vi "display_subVI.vi"(11 "input cluster":T2={"path to binary file"=path "C:/Users/Lenovo/Desktop/szakdoga/data", "Start Cursor"=timestamp(0 s since 1904-01-01), "Sec"=60.0, "crossing level"=0.0, "threshold"=0.35, "avg window size"=5, "peak detect width"=30, "invert"=FALSE, "SNR window width [Hz]"=0.5, "felharmonikus N"=2, "End cursor"=timestamp(0 s since 1904-01-01)} {"peak detect width" min=3; "threshold" format="%0.2f"}) -> (3 "data cluster":T1)   [LabVIEW 2019]
uses:
  <vilib>/Waveform/WDTOps.llb/WDT Get Waveform Subset DBL.vi
  <vilib>/Analysis/NI_AALBase.lvlib
  <vilib>/Analysis/1siggen.llb/Ramp Pattern by Samples.vi
  <vilib>/Analysis/1siggen.llb/Ramp Pattern by Delta.vi
panel:
  out "Z axis SNR":cluster{"Ramp Pattern":dbl[], dbl[]}[](graph)
  out "Y axis SNR":cluster{"Ramp Pattern":dbl[], dbl[]}[](graph)
  out "X axis SNR":cluster{"Ramp Pattern":dbl[], dbl[]}[](graph)
  out "resultant SNR":cluster{"Ramp Pattern":dbl[], dbl[]}[](graph)
  out "SNR":dbl
  out "csapás impulzus":cluster{"Ramp Pattern":dbl[], dbl[]}(graph)
  out "csapásszám":cluster{"Ramp Pattern":dbl[], dbl[]}[](graph)
  in  "felbontás [s]":dbl=20.0
  out "freq [Hz]":dbl
  out "PSD":cluster{"f0":dbl, "df":dbl, "magnitude":dbl[]}[](graph)
  out "inspection":cluster{"Y":dbl[], "Y":dbl[]}[](graph)
  out "inspected section":waveform(dbl)[](graph)
  out "read in data":waveform(dbl)[](graph)
  # "30mp-es ablakokkal számított SNR meta adatok"
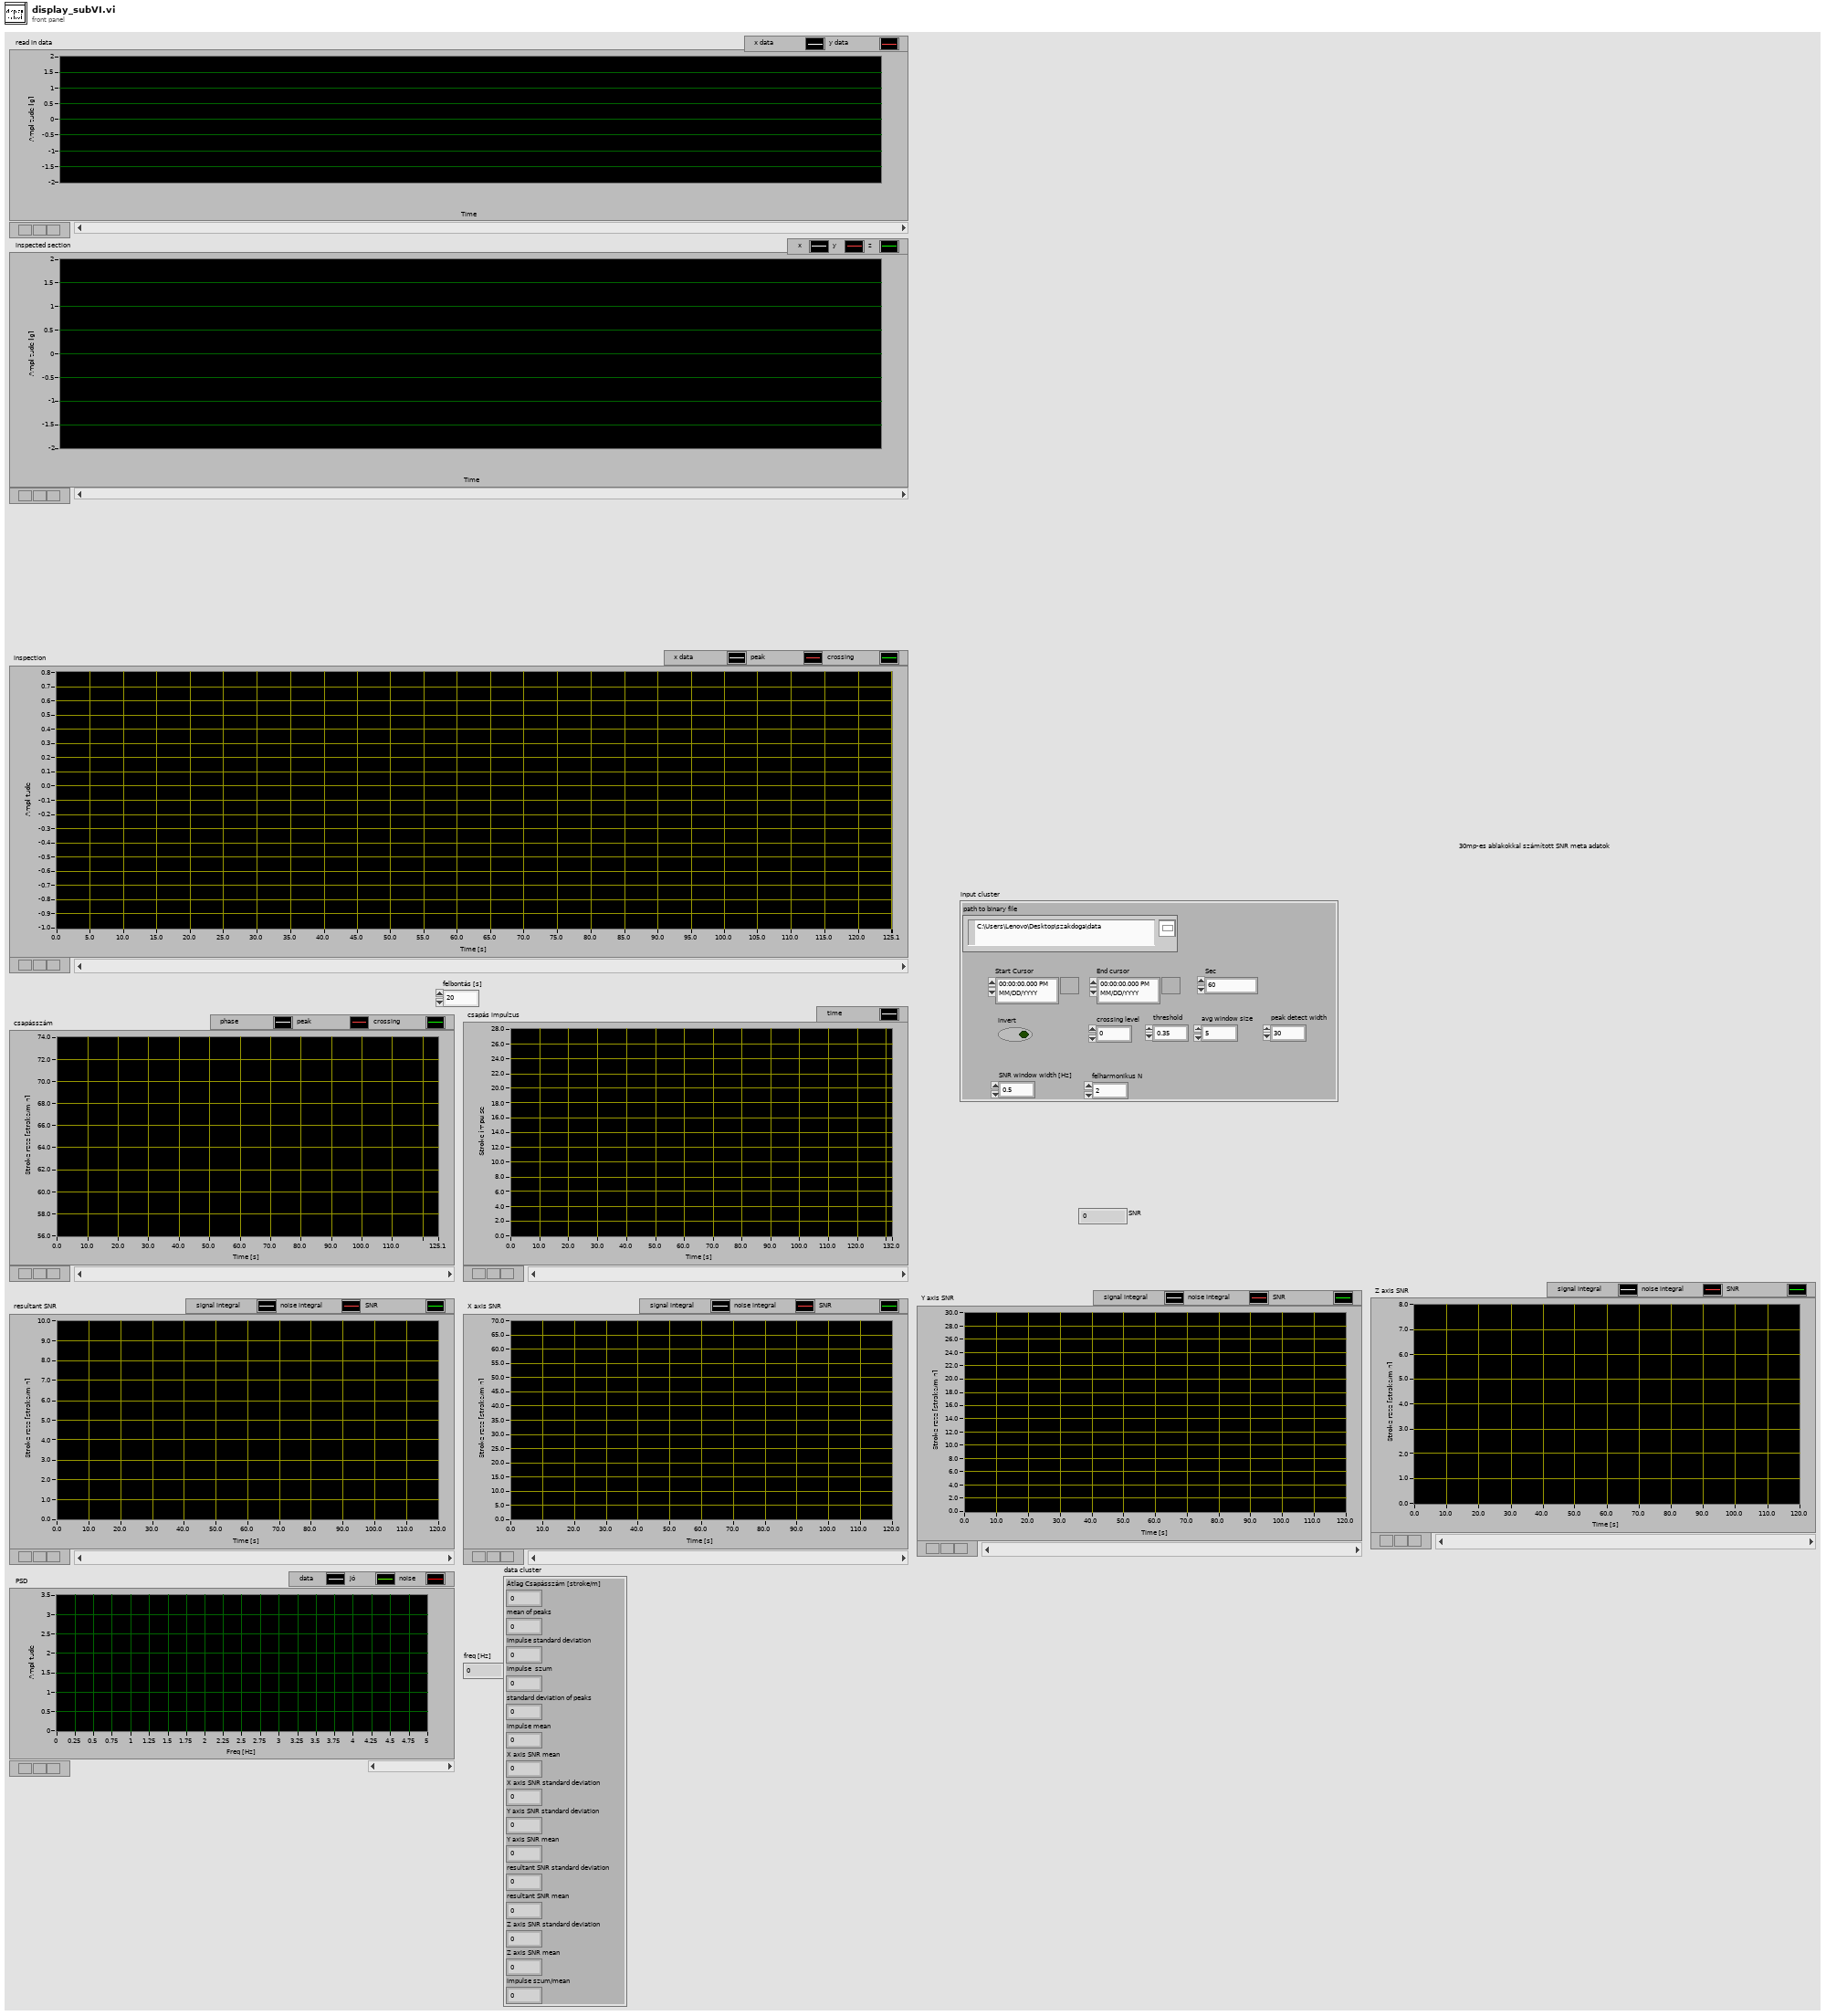
[diagram p1: front panel]
types:
  T1 = cluster{"Átlag Csapásszám [stroke/m]":dbl, "mean of peaks":dbl, "impulse standard deviation":dbl, "impulse  szum":dbl, "standard deviation of peaks":dbl, "impulse mean":dbl, "X axis SNR mean":dbl, "X axis SNR standard deviation":dbl, "Y axis SNR standard deviation":dbl, "Y axis SNR mean":dbl, "resultant SNR standard deviation":dbl, "resultant SNR mean":dbl, "Z axis SNR standard deviation":dbl, "Z axis SNR mean":dbl, "impulse szum/mean":dbl}
  T2 = cluster{"path to binary file":path, "Start Cursor":timestamp, "Sec":dbl, "crossing level":dbl, "threshold":dbl, "avg window size":i32, "peak detect width":i32, "invert":bool, "SNR window width [Hz]":dbl, "felharmonikus N":i32, "End cursor":timestamp}
  T3 = typedef "control_time_informations.ctl" = cluster{"starting time":timestamp, "ending time":timestamp, "dt[s]":dbl, "sampling rate [Hz]":dbl, "length":dbl}
  T4 = typedef "control_all_in_one_package.ctl" = cluster{"memory structure":T5, "actigraph settings":T6, "time informations":T3, "measurement data":T7}
  T5 = typedef "control_memory_structure.ctl" = cluster{"length of metadata [byte]":i32, "length of page [byte]":i32, "length of measurement data on page [byte]":i32, "length of dataset [byte]":i32}
  T6 = typedef "control_measurement_settings.ctl" = cluster{"sampling frequency [Hz]":dbl, "measurement interval [± g]":i32, "high precision?":bool, "number of pages":i32, "rate code":i32, "range code":i32, "id":i32}
  T7 = typedef "control_measurement_data.ctl" = cluster{"number of samples per axis":i32, "timestamp array":dbl[], "offset array":dbl[], "x, y, z axis data":waveform(dbl)[], "normalised magnitude of acceleartion vectors":waveform(dbl), "calibration coefficients":T8, "statistics":T9, "battery voltage":waveform(dbl), "magnitude of acceleartion vectors":waveform(dbl)}
  T8 = typedef "control_calibration_coefficients.ctl" = cluster{"Sx":dbl, "Ox":dbl, "Sy":dbl, "Oy":dbl, "Sz":dbl, "Oz":dbl}
  T9 = typedef "control_statistics.ctl" = cluster{"mean of x axis acceleration":dbl, "standard devation of x axis acceleration":dbl, "mean of y axis acceleration":dbl, "standard devation of y axis acceleration":dbl, "mean of z axis acceleration":dbl, "standard devation of z axis acceleration":dbl, "mean of normalised magnitude of acceleration":dbl, "standard devation of normalised magnitude of acceleration":dbl}
  T10 = cluster{"Ramp Pattern":dbl[], "stroke rate":dbl[]}
  T11 = cluster{"Ramp Pattern":dbl[], "stroke rate":dbl[]}[]
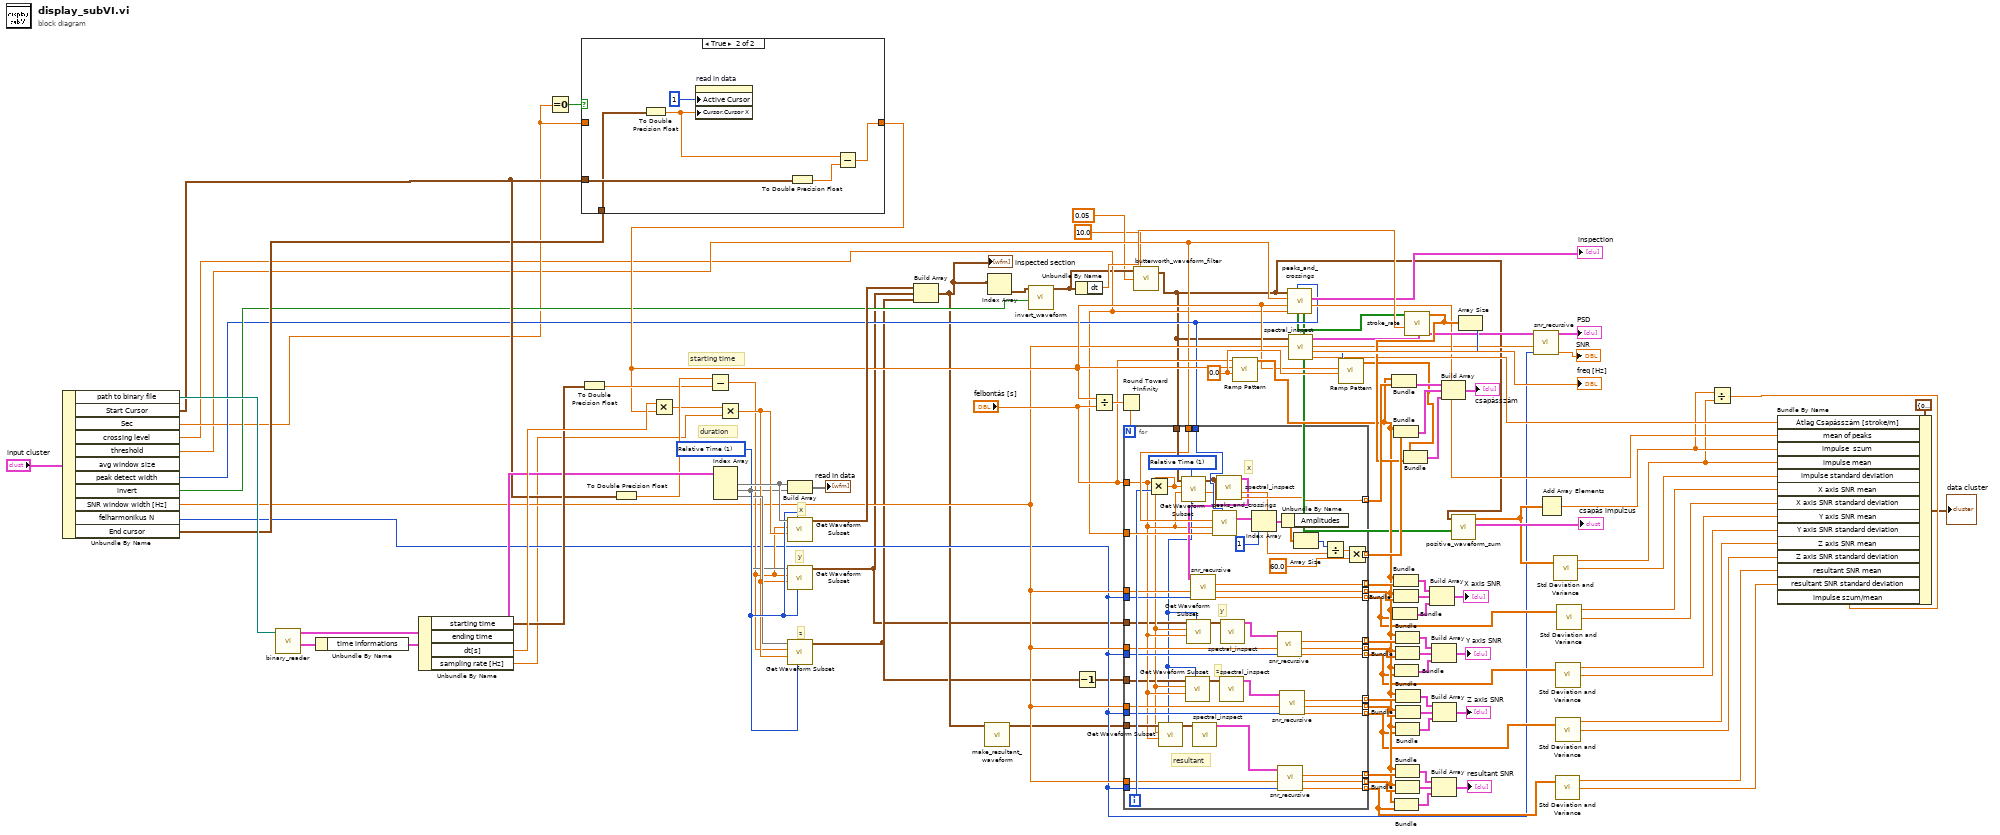
[diagram p0: block diagram]
diagram:
  w82 = 0.0 ("start")
  w101 = u16 1 items=["Samples", "Relative Time"] ("start/duration format")
  # "duration"
  # "starting time"
  # "z"
  # "y"
  # "x"
  n1 = Unbundle By Name("input cluster") -> ("path to binary file"=w27:path, "Start Cursor"=w26:timestamp, "Sec"=w20:dbl, "crossing level"=w16:dbl, "threshold"=w19:dbl, "peak detect width"=w21:i32, "invert"=w24:bool, "SNR window width [Hz]"=w23:dbl, "felharmonikus N"=w22:i32, "End cursor"=w25:timestamp)  [unwired: 1 out]
  n2 = call "binary_reader.vi"("path to binary file"=w27) -> ("time informations"=w105:T3, "all in one package"=w104:T4)  [unwired: 7 in, 1 out]
  n3 = Unbundle By Name(w105) -> ("time informations"=w108:T3)
  n4 = Unbundle By Name(w108) -> ("starting time"=w106:timestamp, "dt[s]"=w107:dbl, "sampling rate [Hz]"=w9:dbl)  [unwired: 1 out]
  n5 = Equal To 0?(x=w20) -> (x = 0?=w46:bool)
  n6 = case shown="True" w46 {
    tunnel: [w109 w113] -> w45
    tunnel: w20 -> [w109 _]
    tunnel: w26 -> [_ w112]
    tunnel: w25 -> [_ w111]
    frame False {
    }
    frame True {
      n7 = To Double Precision Float(number=w111) -> (double precision float=w110:dbl)
      n8 = property on="read in data" class="WFGraph (strict)"("Active Cursor"=1, "Cursor.Cursor X"=w110) -> ()  [unwired: 2 in, 2 out]
      n9 = To Double Precision Float(number=w112) -> (double precision float=w114:dbl)
      n10 = Subtract(x=w110, y=w114) -> (x-y=w113:dbl)
    }
  }
  n11 = To Double Precision Float(number=w106) -> (double precision float=w96:dbl)
  n12 = To Double Precision Float(number=w26) -> (double precision float=w97:dbl)
  n13 = Multiply(x=w107, y=w45) -> (x*y=w10:dbl)
  n14 = Subtract(x=w97, y=w96) -> (x-y=w95:dbl)
  n15 = Index Array(array=w104) -> (element #1=w102, element #2=w98, element #3=w100)  [unwired: 3 in]
  n16 = Multiply(x=w10, y=w9) -> (x*y=w99:dbl)
  n17 = Build Array(w102, w98) -> (→"read in data":void[])
  n18 = call-poly <vilib>:"Get Waveform Subset.vi"("start/duration format"=w101, "duration"=w99, "start samples/time"=w95, "waveform in"=w102) -> ("waveform out"=w94:waveform(dbl))  [unwired: 2 in, 3 out]
  n19 = call-poly <vilib>:"Get Waveform Subset.vi"("start/duration format"=w101, "duration"=w99, "start samples/time"=w95, "waveform in"=w98) -> ("waveform out"=w11:waveform(dbl))  [unwired: 2 in, 3 out]
  n20 = call-poly <vilib>:"Get Waveform Subset.vi"("start/duration format"=w101, "duration"=w99, "start samples/time"=w95, "waveform in"=w100) -> ("waveform out"=w12:waveform(dbl))  [unwired: 2 in, 3 out]
  n21 = Build Array(w94, w11, w12) -> (w14:waveform(dbl)[])
  "inspected section" <- w14
  n22 = call "make_resultant_waveform.vi"("waveform array"=w14) -> ("inspected resultant"=w15:waveform(dbl))  [unwired: 10 in]
  n23 = Index Array(array=w14) -> (element=w85:waveform(dbl))  [unwired: 1 in]
  n24 = call "invert_waveform.vi"("invert"=w24, "waveform"=w85) -> ("output waveform"=w4:waveform(dbl))  [unwired: 9 in]
  n25 = Unbundle By Name(w4) -> ("dt"=w83:dbl)
  n26 = Decrement(x=w12) -> (x-1=w13:waveform(dbl))
  n27 = Divide(x=w45, y="felbontás [s]") -> (x/y=w91:dbl)
  n28 = Round Toward +Infinity(x=w91) -> (ceil(x): smallest int >= x=w92:dbl)
  n29 = call "butterworth_waveform_filter.vi"("high cutoff freq"=10.0, "low cutoff freq"=0.05, "input"=w4) -> ("filtered"=w3:waveform(dbl))  [unwired: 1 in]
  n30 = for {
    N: w92 -> [_]
    tunnel: "felbontás [s]" -> [w120]
    tunnel: w3 -> [w164]
    tunnel: [w163] -> w87 mode=indexing
    tunnel: [w155] -> w86 mode=indexing
    tunnel: w16 -> [w154]
    tunnel: w21 -> [w153]
    tunnel: w19 -> [w152]
    tunnel: w23 -> [w148]
    tunnel: w22 -> [w147]
    tunnel: [w146] -> w75 mode=indexing
    tunnel: [w145] -> w74 mode=indexing
    tunnel: [w144] -> w47 mode=indexing
    tunnel: w23 -> [w140]
    tunnel: w22 -> [w141]
    tunnel: [w138] -> w64 mode=indexing
    tunnel: [w142] -> w65 mode=indexing
    tunnel: [w143] -> w50 mode=indexing
    tunnel: w15 -> [w136]
    tunnel: w23 -> [w133]
    tunnel: w22 -> [w132]
    tunnel: [w134] -> w63 mode=indexing
    tunnel: [w131] -> w62 mode=indexing
    tunnel: [w130] -> w49 mode=indexing
    tunnel: w23 -> [w126]
    tunnel: w22 -> [w127]
    tunnel: [w125] -> w52 mode=indexing
    tunnel: [w128] -> w53 mode=indexing
    tunnel: [w129] -> w48 mode=indexing
    tunnel: w11 -> [w118]
    tunnel: w13 -> [w117]
    i -> [w150]
    w116 = u16 1 items=["Samples", "Relative Time"] ("start/duration format")
    # "resultant"
    # "z"
    # "y"
    # "x"
    n31 = Multiply(x=w120, y=w150) -> (x*y=w119:dbl)
    n32 = call-poly <vilib>:"Get Waveform Subset.vi"("start/duration format"=w116, "duration"=w120, "start samples/time"=w119, "waveform in"=w136) -> ("waveform out"=w137:waveform(dbl))  [unwired: 2 in, 3 out]
    n33 = call-poly <vilib>:"Get Waveform Subset.vi"("start/duration format"=w116, "duration"=w120, "start samples/time"=w119, "waveform in"=w164) -> ("actual duration"=w149:dbl, "waveform out"=w151:waveform(dbl))  [unwired: 2 in, 2 out]
    n34 = call-poly <vilib>:"Get Waveform Subset.vi"("start/duration format"=w116, "duration"=w120, "start samples/time"=w119, "waveform in"=w117) -> ("waveform out"=w124:waveform(dbl))  [unwired: 2 in, 3 out]
    n35 = call-poly <vilib>:"Get Waveform Subset.vi"("start/duration format"=w116, "duration"=w120, "start samples/time"=w119, "waveform in"=w118) -> ("waveform out"=w122:waveform(dbl))  [unwired: 2 in, 3 out]
    n36 = call "spectral_inspect.vi"("waveform"=w137) -> ("PSD"=w135:cluster{"f0":dbl, "df":dbl, "magnitude":dbl[]})  [unwired: 6 in, 4 out]
    n37 = call "peaks_and_crossings.vi"("width"=w153, "crossing level"=w154, "end"=w120, "threshold"=w152, "waveform"=w151) -> ("all in array"=w162:cluster{dbl[], "Amplitudes":dbl[]}[])  [unwired: 6 out]
    n38 = call "spectral_inspect.vi"("waveform"=w151) -> ("Csapásszám [stroke/min]"=w163:dbl, "PSD"=w139:cluster{"f0":dbl, "df":dbl, "magnitude":dbl[]})  [unwired: 6 in, 3 out]
    n39 = call "snr_recursive.vi"("felharmonikus N"=w141, "width [Hz]"=w140, "PSD"=w139) -> ("SNR"=w143:dbl, "Noise Integral"=w142:dbl, "Signal Integral"=w138:dbl)  [unwired: 5 in, 1 out]
    n40 = call "spectral_inspect.vi"("waveform"=w124) -> ("PSD"=w123:cluster{"f0":dbl, "df":dbl, "magnitude":dbl[]})  [unwired: 6 in, 4 out]
    n41 = call "spectral_inspect.vi"("waveform"=w122) -> ("PSD"=w121:cluster{"f0":dbl, "df":dbl, "magnitude":dbl[]})  [unwired: 6 in, 4 out]
    n42 = Index Array(array=w162, index=1) -> (element=w160:cluster{dbl[], "Amplitudes":dbl[]})
    n43 = call "snr_recursive.vi"("felharmonikus N"=w132, "width [Hz]"=w133, "PSD"=w121) -> ("SNR"=w130:dbl, "Noise Integral"=w131:dbl, "Signal Integral"=w134:dbl)  [unwired: 5 in, 1 out]
    n44 = call "snr_recursive.vi"("felharmonikus N"=w147, "width [Hz]"=w148, "PSD"=w135) -> ("SNR"=w144:dbl, "Noise Integral"=w145:dbl, "Signal Integral"=w146:dbl)  [unwired: 5 in, 1 out]
    n45 = call "snr_recursive.vi"("felharmonikus N"=w127, "width [Hz]"=w126, "PSD"=w123) -> ("SNR"=w129:dbl, "Noise Integral"=w128:dbl, "Signal Integral"=w125:dbl)  [unwired: 5 in, 1 out]
    n46 = Unbundle By Name(w160) -> ("Amplitudes"=w159:dbl[])
    n47 = Array Size(array=w159) -> (size(s)=w158:i32)
    n48 = Divide(x=w158, y=w149) -> (x/y=w157:dbl)
    n49 = Multiply(x=w157, y=60.0) -> (x*y=w155:dbl)
  }
  n50 = call-poly <vilib>:"Ramp Pattern.vi"("start"=w82, "end"=w45, "delta"="felbontás [s]") -> ("Ramp Pattern"=w51:dbl[])  [unwired: 6 in, 2 out]
  n51 = call "peaks_and_crossings.vi"("width"=w21, "crossing level"=w16, "end"=w45, "threshold"=w19, "waveform"=w3) -> ("mean of peaks"=w40:dbl, "all in array"=→"inspection":cluster{dbl[], "Amplitudes":dbl[]}[], "plus-minus crossing?"=w17:bool[], "minus-plus crossing?"=w18:bool[])  [unwired: 3 out]
  n52 = call "spectral_inspect.vi"("waveform"=w3) -> ("Csapásszám [stroke/min]"=w41:dbl, "freq"=→"freq [Hz]":dbl, "PSD"=w76:cluster{"f0":dbl, "df":dbl, "magnitude":dbl[]})  [unwired: 6 in, 2 out]
  n53 = Bundle("Ramp Pattern"=w51, w87) -> (w90:cluster{"Ramp Pattern":dbl[], dbl[]})  [unwired: 1 in]
  n54 = Bundle("Ramp Pattern"=w51, w50) -> (w68:cluster{"Ramp Pattern":dbl[], dbl[]})  [unwired: 1 in]
  n55 = Bundle("Ramp Pattern"=w51, w86) -> (w89:cluster{"Ramp Pattern":dbl[], dbl[]})  [unwired: 1 in]
  n56 = Bundle("Ramp Pattern"=w51, w64) -> (w66:cluster{"Ramp Pattern":dbl[], dbl[]})  [unwired: 1 in]
  n57 = Bundle("Ramp Pattern"=w51, w65) -> (w67:cluster{"Ramp Pattern":dbl[], dbl[]})  [unwired: 1 in]
  n58 = Bundle("Ramp Pattern"=w51, w49) -> (w59:cluster{"Ramp Pattern":dbl[], dbl[]})  [unwired: 1 in]
  n59 = Bundle("Ramp Pattern"=w51, w47) -> (w71:cluster{"Ramp Pattern":dbl[], dbl[]})  [unwired: 1 in]
  n60 = Bundle("Ramp Pattern"=w51, w63) -> (w61:cluster{"Ramp Pattern":dbl[], dbl[]})  [unwired: 1 in]
  n61 = Bundle("Ramp Pattern"=w51, w62) -> (w60:cluster{"Ramp Pattern":dbl[], dbl[]})  [unwired: 1 in]
  n62 = Bundle("Ramp Pattern"=w51, w48) -> (w56:cluster{"Ramp Pattern":dbl[], dbl[]})  [unwired: 1 in]
  n63 = Bundle("Ramp Pattern"=w51, w75) -> (w73:cluster{"Ramp Pattern":dbl[], dbl[]})  [unwired: 1 in]
  n64 = Bundle("Ramp Pattern"=w51, w74) -> (w72:cluster{"Ramp Pattern":dbl[], dbl[]})  [unwired: 1 in]
  n65 = Bundle("Ramp Pattern"=w51, w52) -> (w54:cluster{"Ramp Pattern":dbl[], dbl[]})  [unwired: 1 in]
  n66 = Bundle("Ramp Pattern"=w51, w53) -> (w55:cluster{"Ramp Pattern":dbl[], dbl[]})  [unwired: 1 in]
  n67 = call "stroke_rate.vi"("dt"=w83, "minus-plus"=w18) -> ("stroke rate"=w80:dbl[])  [unwired: 9 in]
  n68 = Build Array(w66, w67, w68) -> (→"X axis SNR":cluster{"Ramp Pattern":dbl[], dbl[]}[])
  n69 = Build Array(w61, w60, w59) -> (→"Y axis SNR":cluster{"Ramp Pattern":dbl[], dbl[]}[])
  n70 = Build Array(w73, w72, w71) -> (→"resultant SNR":cluster{"Ramp Pattern":dbl[], dbl[]}[])
  n71 = Build Array(w54, w55, w56) -> (→"Z axis SNR":cluster{"Ramp Pattern":dbl[], dbl[]}[])
  n72 = call "positive_waveform_sum.vi"("plus-minus"=w17, "waveform"=w3) -> ("csapás impulzus"=→"csapás impulzus":cluster{"Ramp Pattern":dbl[], dbl[]}, "Integral X"=w77:dbl[])  [unwired: 8 in]
  n73 = Array Size(array=w80) -> (size(s)=w81:i32)
  n74 = call-poly <vilib>:"Ramp Pattern.vi"("start"=w82, "end"=w45, "samples"=w81) -> ("Ramp Pattern"=w78:dbl[])  [unwired: 7 in, 1 out]
  n75 = Bundle("Ramp Pattern"=w78, "stroke rate"=w80) -> (w84:T10)  [unwired: 1 in]
  n76 = Build Array(w90, w89, w84) -> (→"csapásszám":T11)
  n77 = call "snr_recursive.vi"("felharmonikus N"=w22, "width [Hz]"=w23, "PSD"=w76) -> ("SNR"=→"SNR":dbl, "PSD"=→"PSD":cluster{"f0":dbl, "df":dbl, "magnitude":dbl[]}[])  [unwired: 5 in, 2 out]
  n78 = Add Array Elements(numeric array=w77) -> (sum=w8:dbl)
  n79 = call <vilib>:"Std Deviation and Variance.vi"("X"=w77) -> ("mean"=w7:dbl, "standard deviation"=w39:dbl)  [unwired: 1 in, 1 out]
  n80 = call <vilib>:"Std Deviation and Variance.vi"("X"=w47) -> ("mean"=w32:dbl, "standard deviation"=w31:dbl)  [unwired: 1 in, 1 out]
  n81 = call <vilib>:"Std Deviation and Variance.vi"("X"=w49) -> ("mean"=w36:dbl, "standard deviation"=w35:dbl)  [unwired: 1 in, 1 out]
  n82 = call <vilib>:"Std Deviation and Variance.vi"("X"=w48) -> ("mean"=w34:dbl, "standard deviation"=w33:dbl)  [unwired: 1 in, 1 out]
  n83 = call <vilib>:"Std Deviation and Variance.vi"("X"=w50) -> ("mean"=w38:dbl, "standard deviation"=w37:dbl)  [unwired: 1 in, 1 out]
  n84 = Divide(x=w8, y=w7) -> (x/y=w6:dbl)
  n85 = Bundle By Name ("data")(cluster=T1 {"Átlag Csapásszám [stroke/m]"=0.0, "mean of peaks"=0.0, "impulse standard deviation"=0.0, "impulse  szum"=0.0, "standard deviation of peaks"=0.0, "impulse mean"=0.0, "X axis SNR mean"=0.0, "X axis SNR standard deviation"=0.0, "Y axis SNR standard deviation"=0.0, "Y axis SNR mean"=0.0, "resultant SNR standard deviation"=0.0, "resultant SNR mean"=0.0, "Z axis SNR standard deviation"=0.0, "Z axis SNR mean"=0.0, "impulse szum/mean"=0.0} ("input cluster"), "Átlag Csapásszám [stroke/m]"=w41, "mean of peaks"=w40, "impulse  szum"=w8, "impulse mean"=w7, "impulse standard deviation"=w39, "X axis SNR mean"=w38, "X axis SNR standard deviation"=w37, "Y axis SNR mean"=w36, "Y axis SNR standard deviation"=w35, "Z axis SNR mean"=w34, "Z axis SNR standard deviation"=w33, "resultant SNR mean"=w32, "resultant SNR standard deviation"=w31, "impulse szum/mean"=w6) -> (→"data cluster":T1)
